vi "Event Type Convert to Enum.vi"(1 "Event Type":string) -> (0 "Event Type":T1=enum."Initialize Finish")   [LabVIEW 2019, in "Camera Engine Event.lvlib"]
uses:
  Camera Engine Event.lvlib
  Event Type.ctl
panel:
  out "error out":errorcluster
  in  "error in (no error)":errorcluster
  # "Input"
  # "Output"
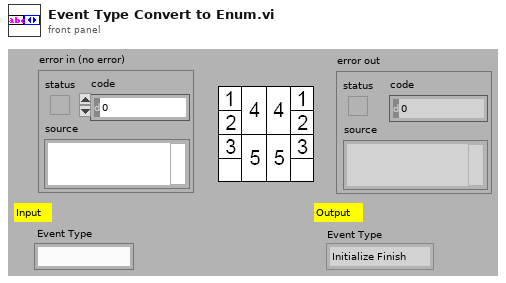
[diagram p1: front panel]
types:
  T1 = typedef "Camera Engine Event.lvlib/Event Type.ctl" = enum16{"Default", "Initialize Finish", "Button 0 Click", "Exit Click", "Exit"}
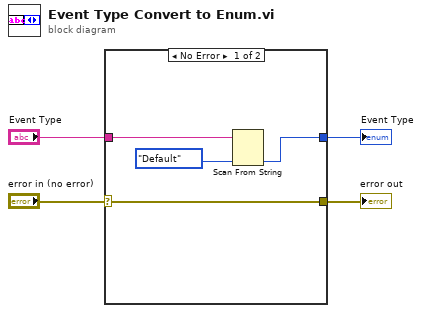
[diagram p0: block diagram]
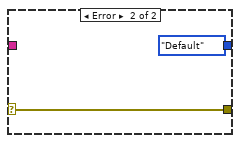
[diagram p2: hidden frame]
diagram:
  n1 = case shown="No Error" "error in (no error)" {
    selector: "error in (no error)" -> [w6 w10]
    tunnel: [w6 w10] -> w2
    tunnel: "Event Type" -> [w8 _]
    tunnel: [w7 Event_Type."Default" ("Event Type")] -> w1
    frame No Error {
      n2 = Scan From String(input string=w8, default 1=Event_Type."Default" ("Event Type")) -> (output 1=w7:T1)  [unwired: 3 in, 3 out]
    }
    frame Error {
    }
  }
  "error out" <- w2
  "Event Type" <- w1
